vi "teleop.vi"(10 "Match Info":T1={"Autonomous Elapsed Seconds"=0.0, "TeleOp Elapsed Seconds"=0.0, "Disabled Elapsed Seconds"=0.0, "Visited Autonomous"=FALSE, "Visited TeleOp"=FALSE, "Visited Disabled"=FALSE, "Autonomous Settings"={"Autonomous Style"=enum."Independent", "VI Refnum"=refnum}}, 11 "Call Context":T2) -> ()   [LabVIEW 2011]
doc: "This VI is called for each TeleOp packet received from the DS where the robot is not disabled. It is often used to read from the joysticks and update I/O or to update setpoints for timed control loops. It should complete and return within 20 milliseconds or it may miss DS packets."
uses:
  <vilib>/Rock Robotics/WPI/DriverStation/WPI_DriverStationDerivedRobotMode.ctl
  <vilib>/Rock Robotics/WPI/DriverStation/WPI_DriverStationMatch Info.ctl
  Robot Global Data.vi
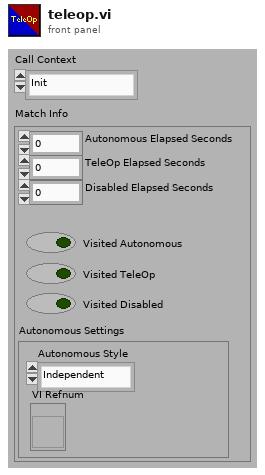
[diagram p1: front panel]
types:
  T1 = typedef "WPI_DriverStationMatch Info.ctl" = cluster{"Autonomous Elapsed Seconds":dbl, "TeleOp Elapsed Seconds":dbl, "Disabled Elapsed Seconds":dbl, "Visited Autonomous":bool, "Visited TeleOp":bool, "Visited Disabled":bool, "Autonomous Settings":cluster{"Autonomous Style":enum16{"Iterative", "Independent"}, "VI Refnum":refnum<vi>}}
  T2 = typedef "WPI_DriverStationDerivedRobotMode.ctl" = enum16{"Init", "Execute", "Stop"}
  T3 = cluster{"Position":cluster{"X":dbl, "Y":dbl}, "Distance (ft)":dbl}[]
  T4 = cluster{"Target Info[0]":cluster{"Position":cluster{"X":dbl, "Y":dbl}, "Distance (ft)":dbl}, "Target Info[1]":cluster{"Position":cluster{"X":dbl, "Y":dbl}, "Distance (ft)":dbl}, "Target Info[2]":cluster{"Position":cluster{"X":dbl, "Y":dbl}, "Distance (ft)":dbl}, "Target Info[3]":cluster{"Position":cluster{"X":dbl, "Y":dbl}, "Distance (ft)":dbl}, "Target Info[4]":cluster{"Position":cluster{"X":dbl, "Y":dbl}, "Distance (ft)":dbl}, "Target Info[5]":cluster{"Position":cluster{"X":dbl, "Y":dbl}, "Distance (ft)":dbl}, "Target Info[6]":cluster{"Position":cluster{"X":dbl, "Y":dbl}, "Distance (ft)":dbl}, "Target Info[7]":cluster{"Position":cluster{"X":dbl, "Y":dbl}, "Distance (ft)":dbl}, "Target Info[8]":cluster{"Position":cluster{"X":dbl, "Y":dbl}, "Distance (ft)":dbl}}
  T5 = typedef "WPI_JoystickDevRef.ctl" = cluster{"Device":T6}
  T6 = typedef "WPI_JoystickDeviceEnum.ctl" = enum16{"USB 1", "USB 2", "USB 3", "USB 4", "Kinect 1", "Kinect 2"}
  T7 = typedef "WPI_JoystickButtonState.ctl" = cluster{"Button 1":bool, "Button 2":bool, "Button 3":bool, "Button 4":bool, "Button 5":bool, "Button 6":bool, "Button 7":bool, "Button 8":bool, "Button 9":bool, "Button 10":bool, "Button 11":bool, "Button 12":bool}
  T8 = cluster{"axis 1 (x)":dbl, "axis 2 (y)":dbl, "axis 3 (throttle)":dbl, "axis 4":dbl, "axis 5":dbl, "axis 6":dbl}
  T9 = typedef "WPI_MotorControlDeviceRef.ctl" = cluster{"DeviceStatus":errorcluster, "Type":enum16{"PWM", "CAN"}, "PWM":cluster{"Digital Module":T10, "PWM Channel":T11, "DeadBand":T12}, "CAN":cluster{"Device Number":u8, "Control Mode":T13, "Semaphore":T14, "Max Vout":dbl}, "Invert":bool, "TransformRef":T15, "InvTransformRef":T15}
  T10 = typedef "FPGA_TypedefDigitalModule.ctl" = enum16{"Digital Module 1", "Digital Module 2"}
  T11 = typedef "FPGA_DIOPWMChannel.ctl" = enum8{"PWM 1", "PWM 2", "PWM 3", "PWM 4", "PWM 5", "PWM 6", "PWM 7", "PWM 8", "PWM 9", "PWM 10", "Invalid"}
  T12 = typedef "WPI_PWMDeadband.ctl" = cluster{"Name":string, "maxPositivePwm":i32, "minPositivePwm":i32, "centerPwm":i32, "maxNegativePwm":i32, "minNegativePwm":i32, "angularRange":u16}
  T13 = typedef "WPI_CANJaguar_ControlMode.ctl" = enum8{"Percent VBus", "Current", "Speed", "Position", "Voltage"}
  T14 = typedef "Semaphore RefNum" = refnum<k1>
  T15 = typedef "WPI_PWMTransform_ConPane.ctl" = refnum<vi>
  T16 = typedef "WPI_RobotDriveDevRef.ctl" = cluster{"DevStatus":errorcluster, "Motors[]":T9[], "Square Inputs":bool, "Max Output":dbl, "Isochronous":bool}
  T17 = typedef "WPI_RelayValue.ctl" = enum16{"Off", "On", "Forward", "Reverse"}
  T18 = typedef "WPI_RelayDevRef.ctl" = cluster{"DevStatus":errorcluster, "Relay Channel":T19, "Digital Module":T10, "Relay Direction":T20}
  T19 = typedef "FPGA_DIORelayChannel.ctl" = enum8{"Relay 1", "Relay 2", "Relay 3", "Relay 4", "Relay 5", "Relay 6", "Relay 7", "Relay 8", "Invalid"}
  T20 = typedef "WPI_RelayDirection.ctl" = enum16{"Both directions", "Forward only", "Reverse only"}
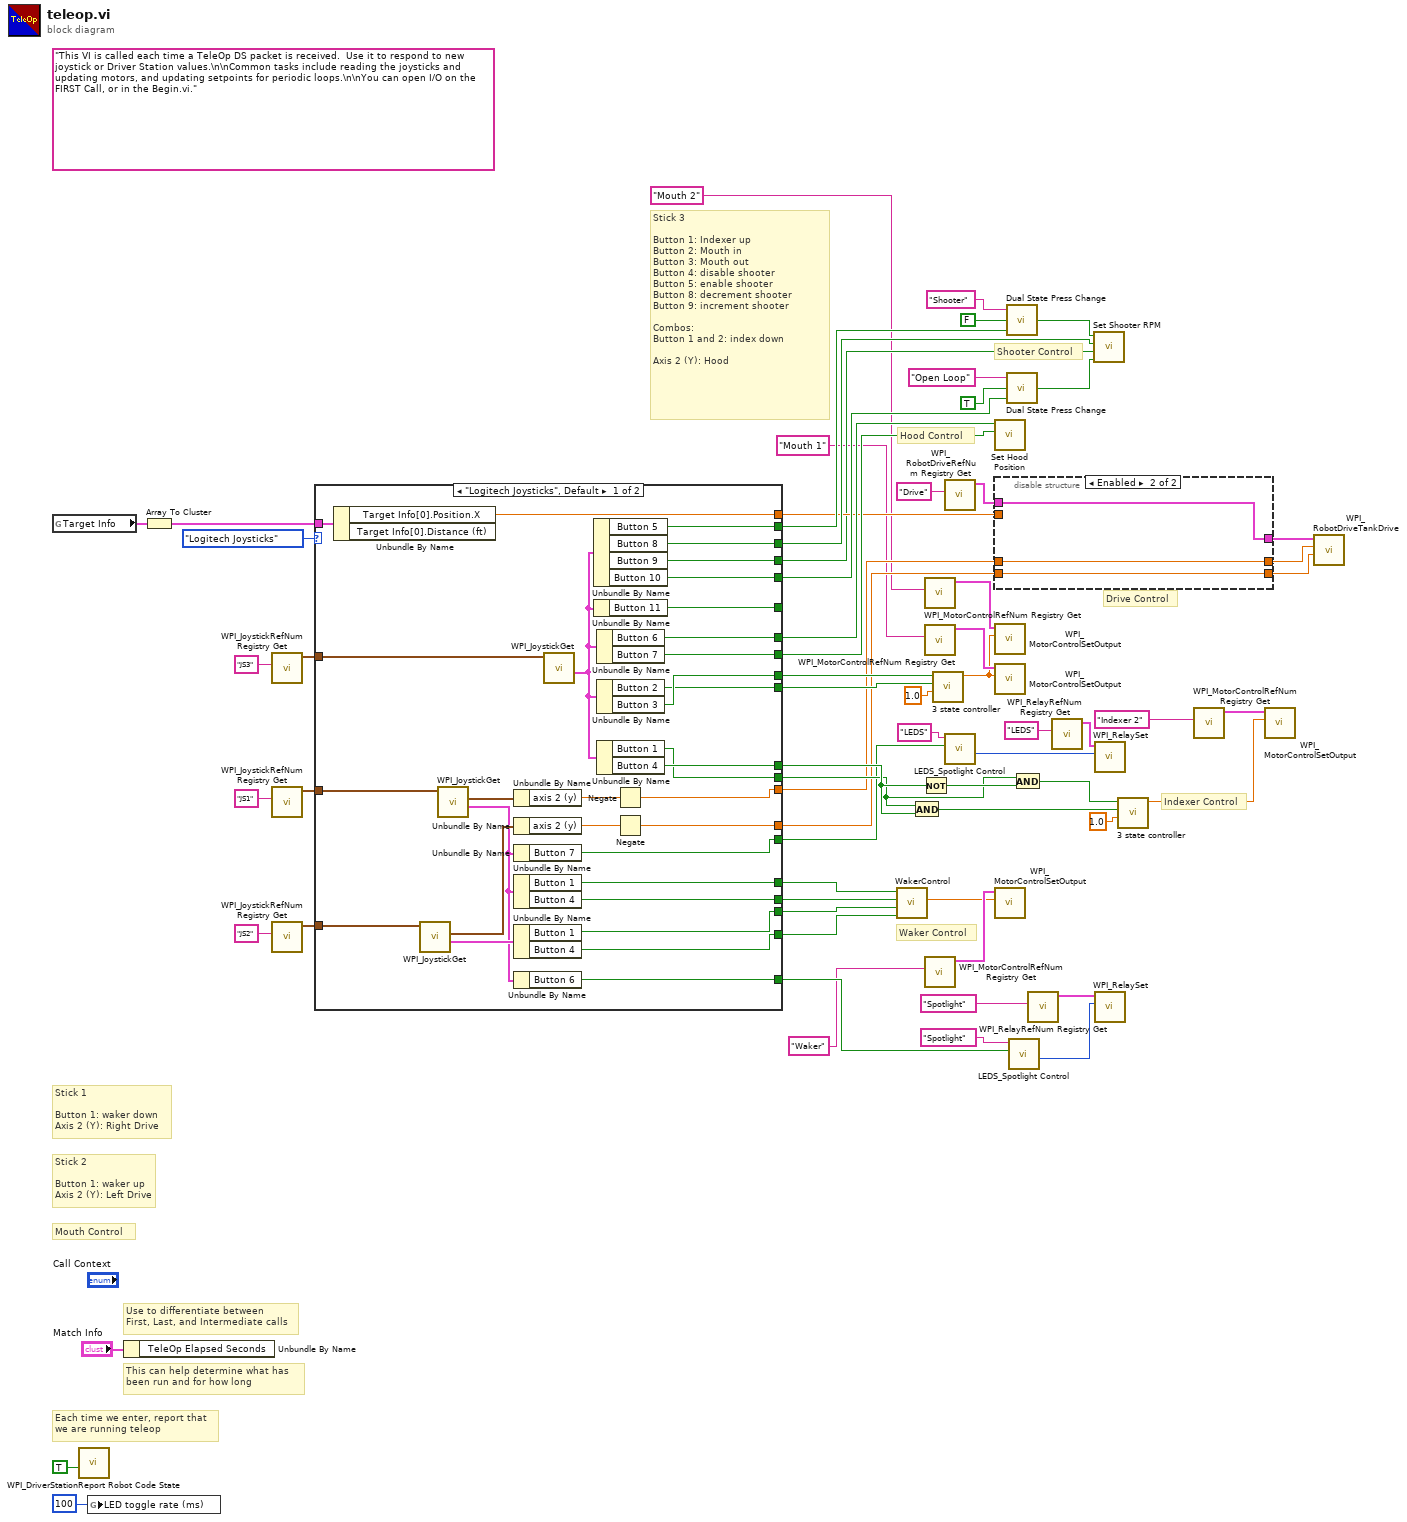
[diagram p0: block diagram]
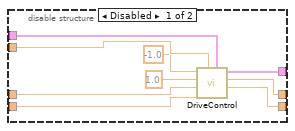
[diagram p2: hidden frame]
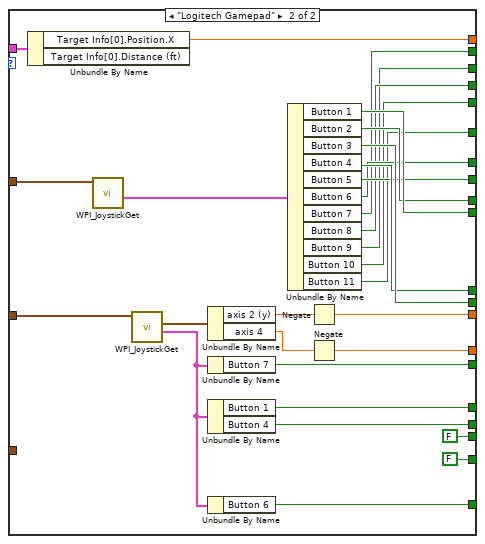
[diagram p3: hidden frame]
diagram:
  (unwired) "This VI is called each time a TeleOp DS packet is received.  Use it to respond to new joystick or Driver Station values.\n\nCommon tasks include reading the joysticks and updating motors, and updating setpoints for periodic loops.\n\nYou can open I/O on the FIRST Call, or in the Begin.vi."
  # "Drive Control"
  # "Shooter Control"
  # "Hood Control"
  # "Indexer Control"
  # "Stick 3\n\nButton 1: Indexer up\nButton 2: Mouth in\nButton 3: Mouth out\nButton 4: disable shooter\nButton 5: enable shooter\nButton 8: decrement shooter\nButton 9: increment shooter\n\nCombos:\nButton 1 and 2: index down\n \nAxis 2 (Y): Hood"
  # "Stick 2\n\nButton 1: waker up\nAxis 2 (Y): Left Drive"
  # "Stick 1\n\nButton 1: waker down\nAxis 2 (Y): Right Drive"
  # "Waker Control"
  # "Mouth Control"
  # "Each time we enter, report that\nwe are running teleop"
  # "Use to differentiate between\nFirst, Last, and Intermediate calls"
  # "This can help determine what has\nbeen run and for how long"
  n1 = global read "Robot Global Data.vi" "Target Info"() -> (w10:T3)
  n2 = call <vilib>:"WPI_DriverStationReport Robot Code State.vi"("TeleOp"=TRUE ("Autonomous")) -> ()  [unwired: 10 in, 1 out]
  n3 = global write "Robot Global Data.vi" "LED toggle rate (ms)"(u32 100 ("LED ms toggle rate")) -> ()
  n4 = Unbundle By Name("Match Info") -> ()  [unwired: 1 out]
  n5 = Array To Cluster(array=w10) -> (cluster=w9:T4)
  n6 = call <vilib>:"WPI_JoystickRefNum Registry Get.vi"("refnum name"="JS3") -> ("JoystickDevRef"=w3:T5)  [unwired: 9 in, 1 out]
  n7 = call <vilib>:"WPI_JoystickRefNum Registry Get.vi"("refnum name"="JS1") -> ("JoystickDevRef"=w6:T5)  [unwired: 9 in, 1 out]
  n8 = call <vilib>:"WPI_JoystickRefNum Registry Get.vi"("refnum name"="JS2") -> ("JoystickDevRef"=w7:T5)  [unwired: 9 in, 1 out]
  n9 = case shown="\"Logitech Joysticks\", Default" enum32{"Logitech Joysticks", "Logitech Gamepad"}."Logitech Joysticks" ("Control Type") {
    tunnel: [w97 w107] -> w62
    tunnel: [w96 w108] -> w59
    tunnel: [w95 w102] -> w43
    tunnel: [w94 w100] -> w42
    tunnel: [w93 w99] -> w41
    tunnel: [w92 w103] -> w40
    tunnel: [w91 w104] -> w39
    tunnel: [w90 w105] -> w38
    tunnel: [w89 w106] -> w37
    tunnel: [w88 w119] -> w35
    tunnel: [w87 w118] -> w34
    tunnel: [w86 w120] -> w31
    tunnel: [w85 w121] -> w28
    tunnel: [w84 FALSE ("Button 1")] -> w26
    tunnel: [w83 FALSE ("Button 4")] -> w25
    tunnel: [w82 w114] -> w21
    tunnel: [w81 w115] -> w20
    tunnel: [w80 w117] -> w19
    tunnel: [w79 w101] -> w18
    tunnel: [w78 w98] -> _
    tunnel: w9 -> [w75 w113]
    tunnel: w7 -> [w74 _]
    tunnel: w6 -> [w73 w122]
    tunnel: w3 -> [w69 w110]
    frame "Logitech Joysticks", Default {
      n10 = Unbundle By Name(w75) -> ("Target Info[0].Position.X"=w82:dbl)  [unwired: 1 out]
      n11 = call <vilib>:"WPI_JoystickGet.vi"("JoystickDevRef"=w74) -> ("Buttons"=w72:T7, "Axes"=w71:T8)  [unwired: 4 in, 1 out]
      n12 = call <vilib>:"WPI_JoystickGet.vi"("JoystickDevRef"=w73) -> ("Buttons"=w68:T7, "Axes"=w70:T8)  [unwired: 4 in, 1 out]
      n13 = Unbundle By Name(w70) -> ("axis 2 (y)"=w76:dbl)
      n14 = Unbundle By Name(w71) -> ("axis 2 (y)"=w77:dbl)
      n15 = Unbundle By Name(w68) -> ("Button 7"=w86:bool)
      n16 = Unbundle By Name(w68) -> ("Button 1"=w88:bool, "Button 4"=w87:bool)
      n17 = Unbundle By Name(w72) -> ("Button 1"=w84:bool, "Button 4"=w83:bool)
      n18 = Unbundle By Name(w68) -> ("Button 6"=w85:bool)
      n19 = call <vilib>:"WPI_JoystickGet.vi"("JoystickDevRef"=w69) -> ("Buttons"=w67:T7)  [unwired: 4 in, 2 out]
      n20 = Unbundle By Name(w67) -> ("Button 5"=w95:bool, "Button 8"=w94:bool, "Button 9"=w79:bool, "Button 10"=w93:bool)
      n21 = Unbundle By Name(w67) -> ("Button 11"=w78:bool)
      n22 = Unbundle By Name(w67) -> ("Button 6"=w92:bool, "Button 7"=w91:bool)
      n23 = Unbundle By Name(w67) -> ("Button 2"=w96:bool, "Button 3"=w97:bool)
      n24 = Unbundle By Name(w67) -> ("Button 1"=w89:bool, "Button 4"=w90:bool)
      n25 = Negate(x=w76) -> (-x=w80:dbl)
      n26 = Negate(x=w77) -> (-x=w81:dbl)
    }
    frame "Logitech Gamepad" {
      n27 = Unbundle By Name(w113) -> ("Target Info[0].Position.X"=w114:dbl)  [unwired: 1 out]
      n28 = call <vilib>:"WPI_JoystickGet.vi"("JoystickDevRef"=w110) -> ("Buttons"=w109:T7)  [unwired: 4 in, 2 out]
      n29 = call <vilib>:"WPI_JoystickGet.vi"("JoystickDevRef"=w122) -> ("Buttons"=w123:T7, "Axes"=w124:T8)  [unwired: 4 in, 1 out]
      n30 = Unbundle By Name(w124) -> ("axis 2 (y)"=w125:dbl, "axis 4"=w116:dbl)
      n31 = Unbundle By Name(w123) -> ("Button 7"=w120:bool)
      n32 = Unbundle By Name(w123) -> ("Button 1"=w119:bool, "Button 4"=w118:bool)
      n33 = Unbundle By Name(w123) -> ("Button 6"=w121:bool)
      n34 = Unbundle By Name(w109) -> ("Button 1"=w108:bool, "Button 2"=w107:bool, "Button 3"=w106:bool, "Button 4"=w105:bool, "Button 5"=w104:bool, "Button 6"=w103:bool, "Button 7"=w102:bool, "Button 8"=w101:bool, "Button 9"=w100:bool, "Button 10"=w99:bool, "Button 11"=w98:bool)
      n35 = Negate(x=w125) -> (-x=w117:dbl)
      n36 = Negate(x=w116) -> (-x=w115:dbl)
    }
  }
  n37 = call "WakerControl.vi"("JS2 Button 4"=w25, "JS2 Button 1"=w26, "JS1 Button 4"=w34, "JS1 Button 1"=w35) -> ("Speed Out"=w33:dbl)  [unwired: 5 in]
  n38 = And(x=w37, y=w38) -> (x .and. y?=w55:bool)
  n39 = Not(x=w38) -> (.not. x?=w44:bool)
  n40 = call <vilib>:"WPI_MotorControlRefNum Registry Get.vi"("refnum name"="Mouth 2") -> ("MotorControlDevRef"=w61:T9)  [unwired: 9 in, 1 out]
  n41 = call <vilib>:"WPI_MotorControlRefNum Registry Get.vi"("refnum name"="Mouth 1") -> ("MotorControlDevRef"=w63:T9)  [unwired: 9 in, 1 out]
  n42 = call <vilib>:"WPI_MotorControlRefNum Registry Get.vi"("refnum name"="Waker") -> ("MotorControlDevRef"=w52:T9)  [unwired: 9 in, 1 out]
  n43 = call "3 state controller.vi"("Power"=1.0, "Backward"=w59, "Forward"=w62) -> ("Numeric"=w60:dbl)  [unwired: 8 in]
  n44 = call <vilib>:"WPI_RobotDriveRefNum Registry Get.vi"("refnum name"="Drive") -> ("RobotDriveDevRef"=w17:T16)  [unwired: 9 in, 1 out]
  n45 = call "LEDS_Spotlight Control.vi"("LEDs or Spotlight"="LEDS", "JS 1 Button 7"=w31) -> ("Relay State"=w32:T17)  [unwired: 8 in]
  n46 = call "Set Hood Position.vi"("Increment"=w39, "Decrement"=w40) -> ()  [unwired: 10 in]
  n47 = disable-structure shown="Enabled" {
    disable-tunnel: [w134 w135] -> w24
    disable-tunnel: [w133 w137] -> w23
    disable-tunnel: [w132 w136] -> w22
    disable-tunnel: w21 -> [w131 _]
    disable-tunnel: w20 -> [w130 w136]
    disable-tunnel: w19 -> [w129 w137]
    disable-tunnel: w17 -> [w128 w135]
    frame Disabled {
      n48 = call "DriveControl.vi"("RobotDriveDevRef"=w128, "Xvalue of Target"=w131, "Right axis value"=w130, "Left axis value"=w129, "Lower Bound"=1.0, "Upper Bound"=-1.0) -> ("Set Right Speed"=w132:dbl, "Set Left Speed"=w133:dbl, "RobotDriveDevRef"=w134:T16)  [unwired: 3 in]
    }
    frame Enabled {
    }
  }
  n49 = call <vilib>:"WPI_MotorControlSetOutput.vi"("Output"=w60, "MotorControlDevRef"=w61) -> ()  [unwired: 8 in, 2 out]
  n50 = call <vilib>:"WPI_MotorControlSetOutput.vi"("Output"=w60, "MotorControlDevRef"=w63) -> ()  [unwired: 8 in, 2 out]
  n51 = call <vilib>:"WPI_MotorControlSetOutput.vi"("Output"=w33, "MotorControlDevRef"=w52) -> ()  [unwired: 8 in, 2 out]
  n52 = call "Dual State Press Change.vi"("Enable/Disable"=w43, "Initial"=FALSE, "Value Name"="Shooter") -> ("Enabled"=w48:bool)
  n53 = call "Dual State Press Change.vi"("Enable/Disable"=w41, "Initial"=TRUE, "Value Name"="Open Loop") -> ("Enabled"=w45:bool)
  n54 = call "LEDS_Spotlight Control.vi"("LEDs or Spotlight"="Spotlight", "JS 1 Button 7"=w28) -> ("Relay State"=w27:T17)  [unwired: 8 in]
  n55 = And(x=w37, y=w44) -> (x .and. y?=w56:bool)
  n56 = call <vilib>:"WPI_RelayRefNum Registry Get.vi"("refnum name"="Spotlight") -> ("RelayDevRef"=w57:T18)  [unwired: 9 in, 1 out]
  n57 = call <vilib>:"WPI_RelayRefNum Registry Get.vi"("refnum name"="LEDS") -> ("RelayDevRef"=w51:T18)  [unwired: 9 in, 1 out]
  n58 = call "Set Shooter RPM.vi"("Open Loop"=w45, "Increment"=w18, "Decrement"=w42, "Shooter Enabled"=w48) -> ()  [unwired: 8 in]
  n59 = call <vilib>:"WPI_RelaySet.vi"("RelayValue"=w32, "RelayDevRef"=w51) -> ()  [unwired: 8 in, 2 out]
  n60 = call <vilib>:"WPI_RelaySet.vi"("RelayValue"=w27, "RelayDevRef"=w57) -> ()  [unwired: 8 in, 2 out]
  n61 = call "3 state controller.vi"("Power"=1.0, "Backward"=w55, "Forward"=w56) -> ("Numeric"=w36:dbl)  [unwired: 8 in]
  n62 = call <vilib>:"WPI_MotorControlRefNum Registry Get.vi"("refnum name"="Indexer 2") -> ("MotorControlDevRef"=w53:T9)  [unwired: 9 in, 1 out]
  n63 = call <vilib>:"WPI_MotorControlSetOutput.vi"("Output"=w36, "MotorControlDevRef"=w53) -> ()  [unwired: 8 in, 2 out]
  n64 = call <vilib>:"WPI_RobotDriveTankDrive.vi"("Right axis value"=w22, "Left axis value"=w23, "RobotDriveDevRef"=w24) -> ()  [unwired: 7 in, 2 out]
